vi "Reopen Files.vi"(8 "error in (no error)":errorcluster, 11 "Frame Grabber Data In":T2={"Camera Session"="", "Frame"=refnum, "AVI Refnum"=refnum, "Codecs"=[], "Frame number"=0, "Tracking File Refnum"=refnum, "Tick Count"=0, "Probe Object"=refnum, "Playback Probe Data"=[], "Rigid Body"={"Position"={"x (mm)"=0.0, "y (mm)"=0.0, "z (mm)"=0.0}, "Orientation"={"Pitch (rad)"=0.0, "Yaw (rad)"=0.0, "Roll (rad)"=0.0}, "Quaternion"={"qx"=0.0, "qy"=0.0, "qz"=0.0, "qw"=0.0}, "Tracked?"=FALSE}, "Total no frames playback"=0, "Video FPS"=0.0, "Camera connected?"=FALSE, "Scene"=refnum, "Cropped Frame"=refnum, "Tracker FPS"=0.0, "Crop ROI"=[], "Presentation Values"=[], "Elapsed time (ms)"=0, "Camera frames playback"=0, "Refnums"={"Live Refnum"=refnum, "Record Refnum"=refnum, "Playback Refnum"=refnum, "Frame Slider Refnum"=refnum, "Pause Refnum"=refnum, "Home Refnum"=refnum, "Set Crop Refnum"=refnum, "Clear Crop Refnum"=refnum, "stop refnum"=refnum, "Playback Rate Refnum"=refnum, "Presentation Refnum"=refnum, "Crop Time Frame Slider Refnum"=refnum, "Cancel Save Refnum"=refnum, "Reverse Playback Refnum"=refnum, "Recording Settings Refnum"=refnum, "Continuous Playback Refnum"=refnum, "Annotation Refnum"=refnum, "Export All Refnum"=refnum, "Export List Refnum"=refnum, "Fill List Refnum"=refnum, "Save Crop Refnum"=refnum, "Skip Forward Refnum"=refnum, "Skip Backward Refnum"=refnum, "Single Annotation Refnum"=refnum, "Load Video Refnum"=refnum, "Set Start Refnum"=refnum, "Set End Refnum"=refnum, "Add to List Refnum"=refnum, "List of Annotations Refnum"=refnum, "Camera Frame Refnum"=refnum, "Load Image Refnum"=refnum, "Saving Refnum"=refnum}, "Dimensions"={"Probe Dimensions"={"Probe Width"=0.0, "Probe Depth"=0.0, "Probe Height"=0.0}, "Room Dimensions"={"Room Width"=0.0, "Room Depth"=0.0, "Room Height"=0.0}}, "Playback Data As Strings"=[], "Cropped Tracking File Refnum"=refnum, "Cropped AVI Refnum"=refnum, "Header"=[], "Total euclidian distance"=0.0, "Annotation File Path"=path "", "Playback File Path"=path "", "Size per frame"=0.0, "Ground Truth File Refnum"=refnum, "Annotation Array"=[], "Annotation TIFFs Folder"=path "", "overwriting open file?"=FALSE, "Image Sequence"=[], "Video/Image Flag"=enum."Playback Video Frame", "Image sequence?"=FALSE, "Image sequence filenames"=[], "Mask"=refnum, "Crop Type"=enum."Rectangle"}) -> (0 "error out":errorcluster, 1 "Playback video path":path, 2 "Annotation List":T1[](array[typedef]) {"Frame Start" min=0}, 3 "Frame Grabber Data Out":T2={"Camera Session"="", "Frame"=refnum, "AVI Refnum"=refnum, "Codecs"=[], "Frame number"=0, "Tracking File Refnum"=refnum, "Tick Count"=0, "Probe Object"=refnum, "Playback Probe Data"=[], "Rigid Body"={"Position"={"x (mm)"=0.0, "y (mm)"=0.0, "z (mm)"=0.0}, "Orientation"={"Pitch (rad)"=0.0, "Yaw (rad)"=0.0, "Roll (rad)"=0.0}, "Quaternion"={"qx"=0.0, "qy"=0.0, "qz"=0.0, "qw"=0.0}, "Tracked?"=FALSE}, "Total no frames playback"=0, "Video FPS"=0.0, "Camera connected?"=FALSE, "Scene"=refnum, "Cropped Frame"=refnum, "Tracker FPS"=0.0, "Crop ROI"=[], "Presentation Values"=[], "Elapsed time (ms)"=0, "Camera frames playback"=0, "Refnums"={"Live Refnum"=refnum, "Record Refnum"=refnum, "Playback Refnum"=refnum, "Frame Slider Refnum"=refnum, "Pause Refnum"=refnum, "Home Refnum"=refnum, "Set Crop Refnum"=refnum, "Clear Crop Refnum"=refnum, "stop refnum"=refnum, "Playback Rate Refnum"=refnum, "Presentation Refnum"=refnum, "Crop Time Frame Slider Refnum"=refnum, "Cancel Save Refnum"=refnum, "Reverse Playback Refnum"=refnum, "Recording Settings Refnum"=refnum, "Continuous Playback Refnum"=refnum, "Annotation Refnum"=refnum, "Export All Refnum"=refnum, "Export List Refnum"=refnum, "Fill List Refnum"=refnum, "Save Crop Refnum"=refnum, "Skip Forward Refnum"=refnum, "Skip Backward Refnum"=refnum, "Single Annotation Refnum"=refnum, "Load Video Refnum"=refnum, "Set Start Refnum"=refnum, "Set End Refnum"=refnum, "Add to List Refnum"=refnum, "List of Annotations Refnum"=refnum, "Camera Frame Refnum"=refnum, "Load Image Refnum"=refnum, "Saving Refnum"=refnum}, "Dimensions"={"Probe Dimensions"={"Probe Width"=0.0, "Probe Depth"=0.0, "Probe Height"=0.0}, "Room Dimensions"={"Room Width"=0.0, "Room Depth"=0.0, "Room Height"=0.0}}, "Playback Data As Strings"=[], "Cropped Tracking File Refnum"=refnum, "Cropped AVI Refnum"=refnum, "Header"=[], "Total euclidian distance"=0.0, "Annotation File Path"=path "", "Playback File Path"=path "", "Size per frame"=0.0, "Ground Truth File Refnum"=refnum, "Annotation Array"=[], "Annotation TIFFs Folder"=path "", "overwriting open file?"=FALSE, "Image Sequence"=[], "Video/Image Flag"=enum."Playback Video Frame", "Image sequence?"=FALSE, "Image sequence filenames"=[], "Mask"=refnum, "Crop Type"=enum."Rectangle"}, 4 "Both exist and open?":bool, 5 "Number of Video Frames":u32, 7 "Number of Tracker Frames":u32)   [LabVIEW 2017]
uses:
  Controls/Frame Grabber Data.ctl
  <vilib>/userdefined/High Color/IMAQdx.ctl
  <vilib>/vision/Image Controls.llb/IMAQ Image.ctl
  <vilib>/vision/Avi.llb/IMAQ AVI2 Refnum.ctl
  Controls/Rigid Body Info.ctl
  Controls/Position.ctl
  Controls/Orientation.ctl
  Controls/Refnums.ctl
  Controls/Recording Settings.ctl
  Controls/Operator Settings.ctl
  Controls/Operator.ctl
  Controls/Patient Settings.ctl
  Controls/Dimensions.ctl
  Controls/Room Dimensions.ctl
  Controls/Crop Video State.ctl
  Controls/Crop Type.ctl
  Controls/Annotation Sequence Details.ctl
  <vilib>/Utility/file.llb/Read Delimited Spreadsheet (string).vi
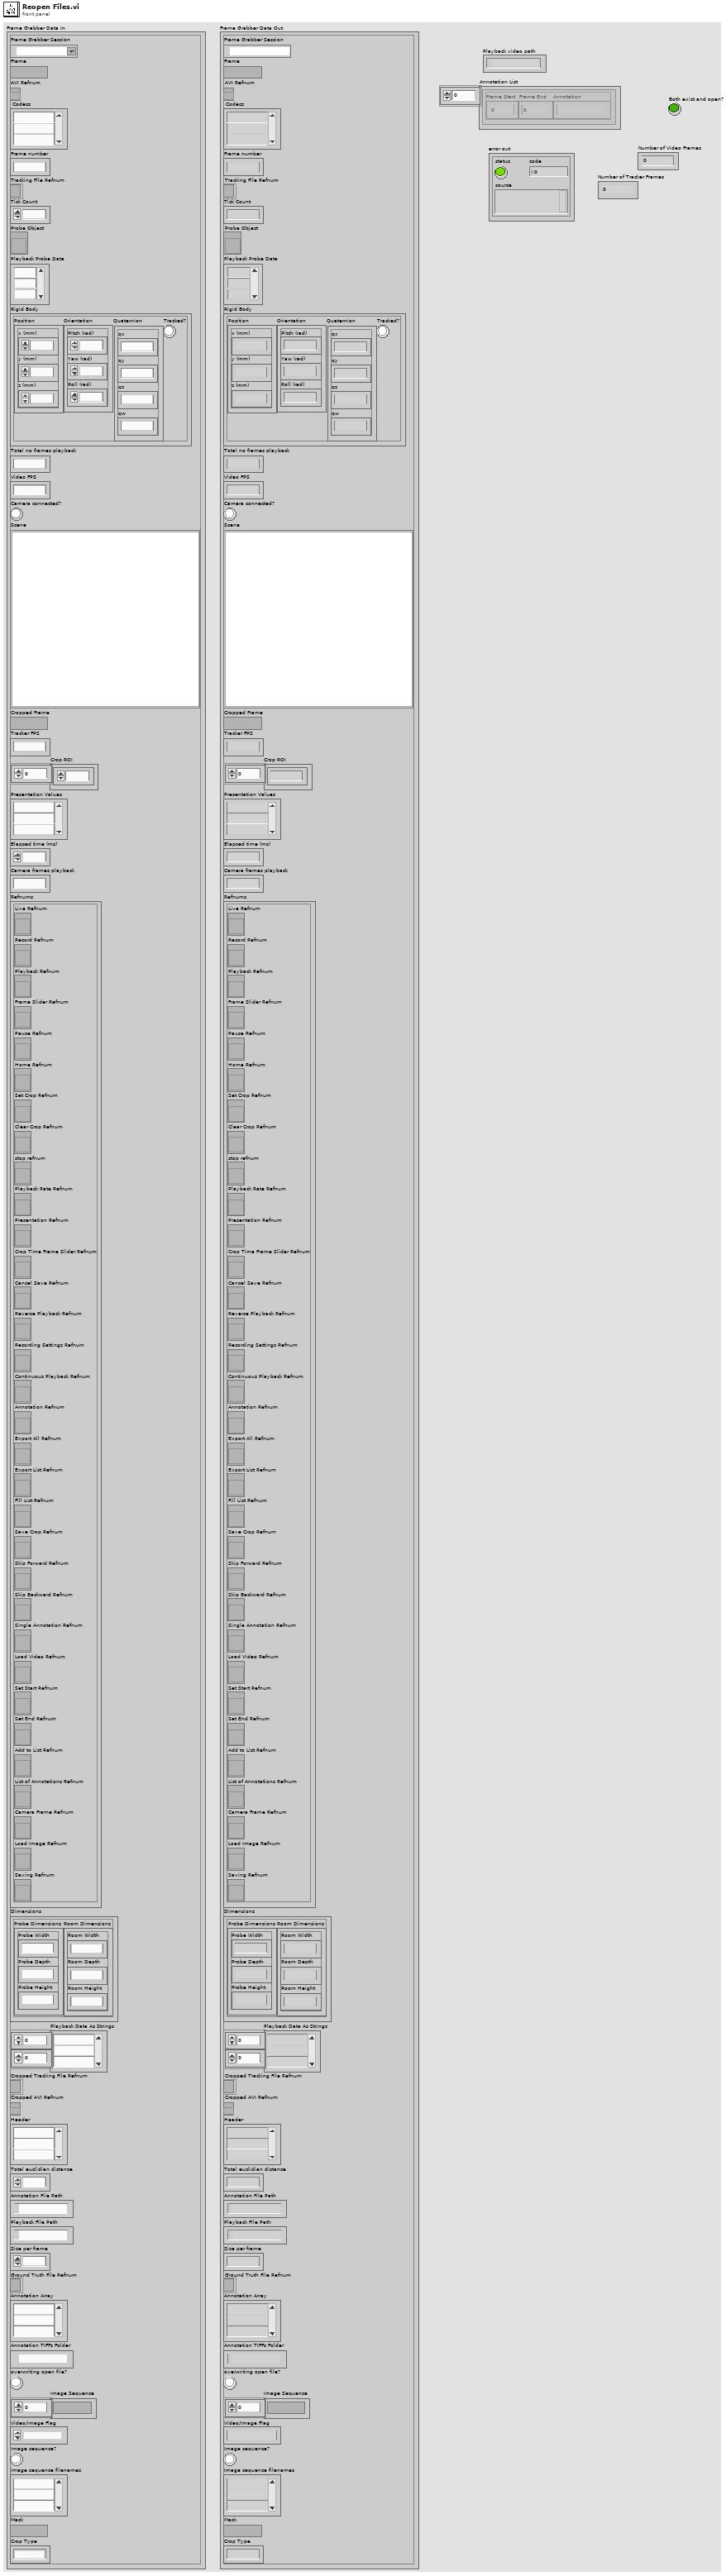
[diagram p1: front panel]
types:
  T1 = typedef "Annotation Sequence Details.ctl" = cluster{"Frame Start":i32, "Frame End":i32, "Annotation":string}
  T2 = typedef "Frame Grabber Data.ctl" = cluster{"Camera Session":T3, "Frame":T4, "AVI Refnum":T5, "Codecs":string[], "Frame number":u32, "Tracking File Refnum":refnum<file>, "Tick Count":u32, "Probe Object":refnum<vi>, "Playback Probe Data":dbl[][], "Rigid Body":T6, "Total no frames playback":i32, "Video FPS":dbl, "Camera connected?":bool, "Scene":refnum<vi>, "Cropped Frame":T4, "Tracker FPS":dbl, "Crop ROI":i32[], "Presentation Values":string[], "Elapsed time (ms)":u32, "Camera frames playback":u32, "Refnums":T9, "Dimensions":T10, "Playback Data As Strings":string[][], "Cropped Tracking File Refnum":refnum<file>, "Cropped AVI Refnum":T5, "Header":string[], "Total euclidian distance":dbl, "Annotation File Path":path, "Playback File Path":path, "Size per frame":dbl, "Ground Truth File Refnum":refnum<file>, "Annotation Array":string[], "Annotation TIFFs Folder":path, "overwriting open file?":bool, "Image Sequence":T4[], "Video/Image Flag":T12, "Image sequence?":bool, "Image sequence filenames":string[], "Mask":T4, "Crop Type":T13}
  T3 = typedef "IMAQdx.ctl" = refnum<k21>
  T4 = typedef "IMAQ Image.ctl" = refnum<image>
  T5 = typedef "IMAQ AVI2 Refnum.ctl" = refnum<k20>
  T6 = typedef "Rigid Body Info.ctl" = cluster{"Position":T7, "Orientation":T8, "Quaternion":cluster{"qx":sgl, "qy":sgl, "qz":sgl, "qw":sgl}, "Tracked?":bool}
  T7 = typedef "Position.ctl" = cluster{"x (mm)":sgl, "y (mm)":sgl, "z (mm)":sgl}
  T8 = typedef "Orientation.ctl" = cluster{"Pitch (rad)":sgl, "Yaw (rad)":sgl, "Roll (rad)":sgl}
  T9 = typedef "Refnums.ctl" = cluster{"Live Refnum":refnum<vi>, "Record Refnum":refnum<vi>, "Playback Refnum":refnum<vi>, "Frame Slider Refnum":refnum<vi>, "Pause Refnum":refnum<vi>, "Home Refnum":refnum<vi>, "Set Crop Refnum":refnum<vi>, "Clear Crop Refnum":refnum<vi>, "stop refnum":refnum<vi>, "Playback Rate Refnum":refnum<vi>, "Presentation Refnum":refnum<vi>, "Crop Time Frame Slider Refnum":refnum<vi>, "Cancel Save Refnum":refnum<vi>, "Reverse Playback Refnum":refnum<vi>, "Recording Settings Refnum":refnum<vi>, "Continuous Playback Refnum":refnum<vi>, "Annotation Refnum":refnum<vi>, "Export All Refnum":refnum<vi>, "Export List Refnum":refnum<vi>, "Fill List Refnum":refnum<vi>, "Save Crop Refnum":refnum<vi>, "Skip Forward Refnum":refnum<vi>, "Skip Backward Refnum":refnum<vi>, "Single Annotation Refnum":refnum<vi>, "Load Video Refnum":refnum<vi>, "Set Start Refnum":refnum<vi>, "Set End Refnum":refnum<vi>, "Add to List Refnum":refnum<vi>, "List of Annotations Refnum":refnum<vi>, "Camera Frame Refnum":refnum<vi>, "Load Image Refnum":refnum<vi>, "Saving Refnum":refnum<vi>}
  T10 = typedef "Dimensions.ctl" = cluster{"Probe Dimensions":cluster{"Probe Width":sgl, "Probe Depth":sgl, "Probe Height":sgl}, "Room Dimensions":T11}
  T11 = typedef "Room Dimensions.ctl" = cluster{"Room Width":dbl, "Room Depth":dbl, "Room Height":dbl}
  T12 = typedef "Crop Video State.ctl" = enum16{"Init", "Wait", "Load Image", "Load Video", "Play/Pause", "Playback Video Frame", "Display Image", "Save Image Sequence", "Save Video", "Export List", "Export All", "Close", "Set Crop Area", "Reset Crop Area", "Crop Inside", "Crop Outside", "Multi-Crop", "Re-Open Files", "Annotate Frame", "Annotate Clip", "Add to List", "Fill List", "Set Start", "Set End", "Error Handling", "Shutdown"}
  T13 = typedef "Crop Type.ctl" = enum16{"Rectangle", "Annulus"}
  T14 = enum8{"Enabled", "Disabled", "Disabled and Grayed Out"}
  T15 = cluster{"Width":u32, "Height":u32, "Frames Per Second":u32, "Codec":string, "Has Data":bool}
  T16 = cluster{"Scale.Range:Minimum":i32, "Number of Frames":u32, "Scale.Range:Minimum":i32}
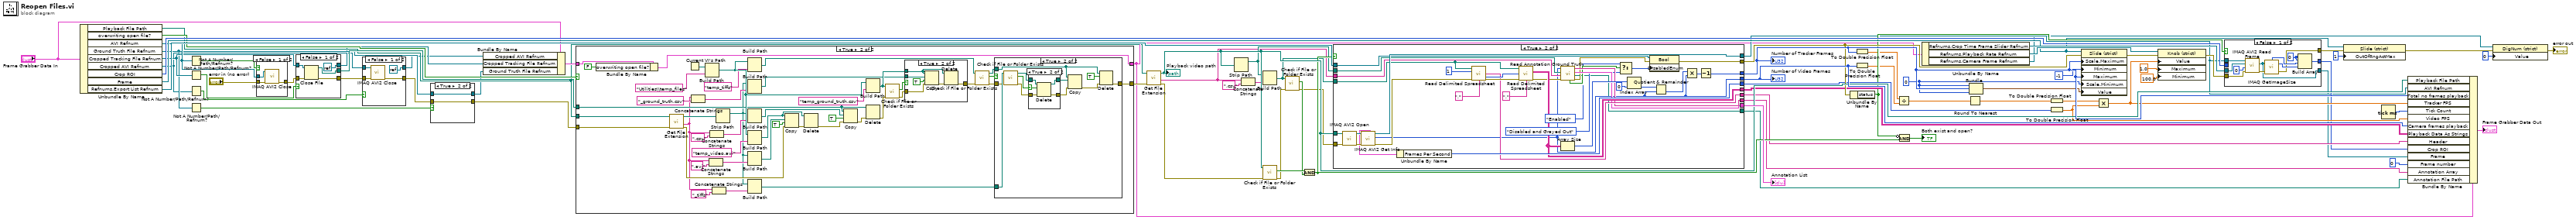
[diagram p0: block diagram]
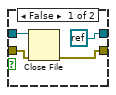
[diagram p2: hidden frame]
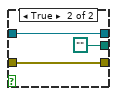
[diagram p4: hidden frame]
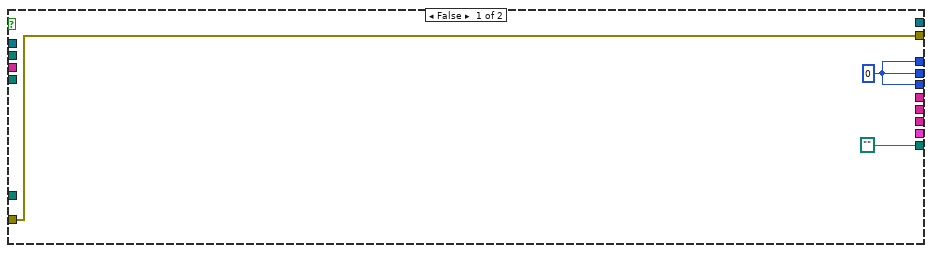
[diagram p7: hidden frame]
diagram:
  w24 = 0 ("Scale.Range:Minimum")
  n1 = Unbundle By Name("Frame Grabber Data In") -> ("Playback File Path"=w6:path, "overwriting open file?"=w7:bool, "AVI Refnum"=w15:T5, "Ground Truth File Refnum"=w5:refnum<file>, "Cropped Tracking File Refnum"=w8:refnum<file>, "Cropped AVI Refnum"=w1:T5, "Crop ROI"=w75:i32[], "Frame"=w76:T4, "Refnums.Export List Refnum"=w77:refnum<vi>)
  n2 = Not A Number/Path/Refnum?(number/path/refnum=w15) -> (NaN/Path/Refnum?=w14:bool)
  n3 = Not A Number/Path/Refnum?(number/path/refnum=w8) -> (NaN/Path/Refnum?=w10:bool)
  n4 = Not A Number/Path/Refnum?(number/path/refnum=w1) -> (NaN/Path/Refnum?=w9:bool)
  n5 = Not A Number/Path/Refnum?(number/path/refnum=w5) -> (NaN/Path/Refnum?=w11:bool)
  n6 = case shown="False" w14 {
    tunnel: [w80 w81] -> w72
    tunnel: "error in (no error)" -> [w79 w81]
    tunnel: w15 -> [w78 _]
    frame False {
      n7 = call "IMAQ AVI2 Close"("error in (no error)"=w79, "AVI Refnum"=w78) -> ("error out"=w80:errorcluster)  [unwired: 9 in]
    }
    frame True {
    }
  }
  n8 = case shown="False" w10 {
    tunnel: w8 -> [w86 w87]
    tunnel: [w85 w89] -> w74
    tunnel: w72 -> [w84 w89]
    tunnel: [w83 path ""] -> w16
    tunnel: [refnum<k0> refnum w87] -> w4
    frame False {
      n9 = Close File(refnum=w86, error in=w84) -> (path=w83:path, error out=w85:errorcluster)
    }
    frame True {
    }
  }
  n10 = case shown="False" w9 {
    tunnel: w1 -> [w93 w94]
    tunnel: w74 -> [w92 w95]
    tunnel: [w91 w95] -> w13
    tunnel: [refnum<k0> refnum w94] -> w3
    frame False {
      n11 = call "IMAQ AVI2 Close"("error in (no error)"=w92, "AVI Refnum"=w93) -> ("error out"=w91:errorcluster)  [unwired: 9 in]
    }
    frame True {
    }
  }
  n12 = case shown="True" w11 {
    tunnel: [w99 w101] -> w12
    tunnel: w13 -> [w98 w101]
    tunnel: w5 -> [w97 w100]
    tunnel: [refnum<k0> refnum w100] -> w2
    frame False {
      n13 = Close File(refnum=w97, error in=w98) -> (error out=w99:errorcluster)  [unwired: 1 out]
    }
    frame True {
    }
  }
  n14 = Bundle By Name(cluster="Frame Grabber Data In", "Cropped AVI Refnum"=w3, "Cropped Tracking File Refnum"=w4, "Ground Truth File Refnum"=w2) -> (w18:T2)
  n15 = case shown="True" w7 {
    tunnel: w18 -> [w103 w147]
    tunnel: [w103 w144] -> w19
    tunnel: [w102 w125] -> w71
    tunnel: w12 -> [w102 w119]
    tunnel: w6 -> [_ w136]
    tunnel: w16 -> [_ w135]
    frame False {
    }
    frame True {
      n16 = Bundle By Name(cluster=w147, "overwriting open file?"=FALSE) -> (w144:T2)
      n17 = call <vilib>:"Get File Extension.vi"("error in (no error)"=w119, "file"=w136) -> ("error out"=w120:errorcluster, "filename without extension"=w106:string, "dup file"=w122:path)  [unwired: 5 in, 2 out]
      n18 = Current VI's Path() -> (path=w142:path)
      n19 = Concatenate Strings(w106, "_ground_truth.csv" ("string")) -> (w111:string)
      n20 = Build Path(base path=w142, name or relative path="Utilities\\temp_files") -> (appended path=w143:path)
      n21 = Concatenate Strings(w106, ".avi" ("string")) -> (w115:string)
      n22 = Concatenate Strings(w106, ".csv" ("string")) -> (w121:string)
      n23 = Concatenate Strings(w106, "_tiffs" ("string")) -> (w107:string)
      n24 = Strip Path(path=w122) -> (stripped path=w105:path)  [unwired: 1 out]
      n25 = Build Path(base path=w143, name or relative path="temp_tiffs") -> (appended path=w133:path)
      n26 = Build Path(base path=w105, name or relative path=w111) -> (appended path=w109:path)
      n27 = Build Path(base path=w105, name or relative path=w121) -> (appended path=w117:path)
      n28 = Build Path(base path=w143, name or relative path="temp_video.avi") -> (appended path=w118:path)
      n29 = Build Path(base path=w105, name or relative path=w115) -> (appended path=w114:path)
      n30 = Build Path(base path=w105, name or relative path=w107) -> (appended path=w104:path)
      n31 = Copy(8:w120, 9:TRUE ("overwrite (F)"), 10:w114, 11:w118) -> (0:w134:errorcluster)  [unwired: 1 in, 2 out]
      n32 = Delete(path (use dialog)=w118, error in=w134) -> (error out=w132:errorcluster)  [unwired: 3 in, 2 out]
      n33 = Copy(8:w132, 9:TRUE ("overwrite (F)"), 10:w117, 11:w135) -> (0:w145:errorcluster)  [unwired: 1 in, 2 out]
      n34 = Build Path(base path=w143, name or relative path="temp_ground_truth.csv") -> (appended path=w129:path)
      n35 = Delete(path (use dialog)=w135, error in=w145) -> (error out=w131:errorcluster)  [unwired: 3 in, 2 out]
      n36 = call <vilib>:"Check if File or Folder Exists.vi"("error in (no error)"=w131, "path"=w129) -> ("error out"=w130:errorcluster, "file or folder exists?"=w128:bool)  [unwired: 7 in, 1 out]
      n37 = case shown="True" w128 {
        tunnel: w130 -> [w167 w173]
        tunnel: w129 -> [_ w170]
        tunnel: [w167 w171] -> w127
        tunnel: w109 -> [_ w168]
        frame False {
        }
        frame True {
          n38 = Copy(8:w173, 9:TRUE ("overwrite (F)"), 10:w168, 11:w170) -> (0:w172:errorcluster)  [unwired: 1 in, 2 out]
          n39 = Delete(path (use dialog)=w170, error in=w172) -> (error out=w171:errorcluster)  [unwired: 3 in, 2 out]
        }
      }
      n40 = call <vilib>:"Check if File or Folder Exists.vi"("error in (no error)"=w127, "path"=w133) -> ("error out"=w126:errorcluster, "file or folder exists?"=w124:bool, "dup path"=w123:path)  [unwired: 7 in]
      n41 = case shown="True" w124 {
        tunnel: w126 -> [w148 w154]
        tunnel: w123 -> [_ w157]
        tunnel: [w148 w158] -> w125
        tunnel: w104 -> [_ w155]
        frame False {
        }
        frame True {
          n42 = call <vilib>:"Check if File or Folder Exists.vi"("error in (no error)"=w154, "path"=w155) -> ("error out"=w153:errorcluster, "file or folder exists?"=w152:bool, "dup path"=w151:path)  [unwired: 7 in]
          n43 = case shown="True" w152 {
            selector: w152 -> [_ w165]
            tunnel: w153 -> [w161 w166]
            tunnel: w151 -> [w160 w164]
            tunnel: [w161 w163] -> w150
            tunnel: [w160 w162] -> w149
            frame False {
            }
            frame True {
              n44 = Delete(path (use dialog)=w164, entire hierarchy (F)=w165, error in=w166) -> (deleted path=w162:path, error out=w163:errorcluster)  [unwired: 2 in, 1 out]
            }
          }
          n45 = Copy(8:w150, 10:w149, 11:w157) -> (0:w159:errorcluster)  [unwired: 2 in, 2 out]
          n46 = Delete(path (use dialog)=w157, entire hierarchy (F)=TRUE, error in=w159) -> (error out=w158:errorcluster)  [unwired: 2 in, 2 out]
        }
      }
    }
  }
  n47 = call <vilib>:"Get File Extension.vi"("error in (no error)"=w71, "file"=w6) -> ("error out"=w58:errorcluster, "filename without extension"=w25:string, "dup file"=w64:path)  [unwired: 5 in, 2 out]
  "Playback video path" <- w64
  n48 = Strip Path(path=w64) -> (stripped path=w26:path)  [unwired: 1 out]
  n49 = Concatenate Strings(w25, ".csv" ("string")) -> (w20:string)
  n50 = Build Path(base path=w26, name or relative path=w20) -> (appended path=w56:path)
  n51 = call <vilib>:"Check if File or Folder Exists.vi"("error in (no error)"=w58, "path"=w64) -> ("error out"=w54:errorcluster, "file or folder exists?"=w57:bool)  [unwired: 7 in, 1 out]
  n52 = call <vilib>:"Check if File or Folder Exists.vi"("error in (no error)"=w54, "path"=w56) -> ("error out"=w28:errorcluster, "file or folder exists?"=w55:bool)  [unwired: 7 in, 1 out]
  n53 = And(x=w57, y=w55) -> (x .and. y?=w63:bool)
  n54 = case shown="True" w63 {
    tunnel: w28 -> [w176 w191]
    tunnel: w64 -> [_ w212]
    tunnel: [w176 w182] -> w61
    tunnel: [_ w209] -> w40
    tunnel: w56 -> [_ w204]
    tunnel: [w175 w187] -> w67
    tunnel: [w175 w207] -> w59
    tunnel: [w175 w185] -> w69
    tunnel: [_ w201] -> w45
    tunnel: [_ w197] -> w44
    tunnel: [_ w195] -> w70
    tunnel: [_ w194] -> w27
    tunnel: w26 -> [_ w193]
    tunnel: w25 -> [_ w192]
    tunnel: w77 -> [_ w184]
    tunnel: [path "" w177] -> w22
    frame False {
      w175 = 0 ("Number of Frames")
    }
    frame True {
      n55 = call "IMAQ AVI2 Open"("error in (no error)"=w191, "AVI File Path"=w212) -> ("error out"=w211:errorcluster, "AVI Refnum"=w210:T5)  [unwired: 8 in]
      n56 = call "IMAQ AVI2 Get Info"("error in (no error)"=w211, "AVI Refnum"=w210) -> ("error out"=w206:errorcluster, "Number of Frames"=w187:u32, "AVI Refnum (duplicate)"=w209:T5, "Frame Data"=w208:T15)  [unwired: 5 in, 1 out]
      n57 = Unbundle By Name(w208) -> ("Frames Per Second"=w207:u32)
      n58 = call-poly <vilib>:"Read Delimited Spreadsheet.vi"("file path (dialog if empty)"=w204, "number of rows (all:-1)"=1, "error in (no error)"=w206, "delimiter (\\t)"="," ("delimiter (\\t)")) -> ("first row"=w197:string[], "mark after read (chars.)"=w202:i32, "error out"=w203:errorcluster)  [unwired: 6 in, 3 out]
      n59 = call-poly <vilib>:"Read Delimited Spreadsheet.vi"("file path (dialog if empty)"=w204, "start of read offset (chars.:0)"=w202, "error in (no error)"=w203, "delimiter (\\t)"="," ("delimiter (\\t)")) -> ("all rows"=w201:string[][], "error out"=w190:errorcluster)  [unwired: 6 in, 4 out]
      n60 = Array Size(array=w201) -> (size(s)=w200:i32[])
      n61 = call "Read Annotation Ground Truth.vi"("Error In"=w190, "Filename without extension"=w192, "Folder"=w193, "Total no frames playback"=w187) -> ("Error Out"=w183:errorcluster, "annotation file path"=w177:path, "Annotation List"=w195:T1[], "Annotation array (strings)"=w194:string[], "annotation list exists?"=w181:bool)  [unwired: 3 in]
      n62 = Select(t=T14."Enabled" ("Disabled"), s=w181, f=T14."Disabled and Grayed Out") -> (s? t:f=w179:T14)
      n63 = Index Array(array=w200, index=0) -> (element=w189:i32)
      n64 = property class="Bool"(reference=w184, error in=w183, "DisabledEnum"=w179) -> (error out=w182:errorcluster)  [unwired: 1 out]
      n65 = Quotient & Remainder(x=w189, y=w187) -> (floor(x/y)=w188:u32)  [unwired: 1 out]
      n66 = Multiply(x=w188, y=w187) -> (x*y=w186:u32)
      n67 = Decrement(x=w186) -> (x-1=w185:u32)
    }
  }
  "Annotation List" <- w70
  "Number of Tracker Frames" <- w69
  "Number of Video Frames" <- w67
  n68 = Unbundle By Name(w61) -> ("status"=w43:bool)
  n69 = To Double Precision Float(number=w69) -> (double precision float=w37:dbl)
  n70 = To Double Precision Float(number=w67) -> (double precision float=w36:dbl)
  n71 = Divide(x=w37, y=w36) -> (x/y=w60:dbl)
  n72 = Compound Arithmetic op=AND(invert w43, w63) -> (→"Both exist and open?":bool)
  n73 = Unbundle By Name(w19) -> ("Refnums.Crop Time Frame Slider Refnum"=w33:refnum<vi>, "Refnums.Playback Rate Refnum"=w53:refnum<vi>, "Refnums.Camera Frame Refnum"=w30:refnum<vi>)
  n74 = Round To Nearest(number=w60) -> (nearest integer value=w38:dbl)
  n75 = Bundle("Scale.Range:Minimum"=w24, "Number of Frames"=w69, "Scale.Range:Minimum"=w24) -> (w46:T16)  [unwired: 1 in]
  n76 = To Double Precision Float(number=w38) -> (double precision float=w47:dbl)
  n77 = To Double Precision Float(number=w59) -> (double precision float=w48:dbl)
  n78 = property class="Slide (strict)"(reference=w33, error in=w61, "Scale.Maximum"=w69, "Minimum"=-1 ("Scale.Range:Minimum"), "Maximum"=w69, "Scale.Minimum"=w24, "Value"=w46) -> (error out=w51:errorcluster)  [unwired: 1 out]
  n79 = Multiply(x=w47, y=w48) -> (x*y=w52:dbl)
  n80 = property class="Knob (strict)"(reference=w53, error in=w51, "Value"=w52, "Maximum"=1.0 ("Data Entry Limits:Maximum"), "Minimum"=100.0 ("Data Entry Limits:Minimum")) -> (error out=w42:errorcluster)  [unwired: 1 out]
  n81 = case shown="False" w43 {
    tunnel: w42 -> [w223 w225]
    tunnel: w75 -> [_ w226]
    tunnel: [w218 w226] -> w41
    tunnel: w40 -> [w217 _]
    tunnel: w76 -> [w215 w224]
    tunnel: [w214 w225] -> w34
    tunnel: [w213 w224] -> w39
    frame False {
      w219 = 0 ("element")
      n82 = call "IMAQ AVI2 Read Frame"("error in (no error)"=w223, "Frame Number"=u32 0, "Image"=w215, "AVI Refnum"=w217) -> ("error out"=w222:errorcluster, "Image Out"=w213:T4)  [unwired: 5 in, 1 out]
      n83 = call "IMAQ GetImageSize"("Image"=w213, "error in (no error)"=w222) -> ("Y Resolution"=w221:i32, "X Resolution"=w220:i32, "error out"=w214:errorcluster)  [unwired: 2 in]
      n84 = Build Array(w219, w219, w220, w221) -> (w218:i32[])
    }
    frame True {
    }
  }
  n85 = property class="Slide (strict)"(reference=w33, error in=w34, "OutOfRngActMax"=u8 1 ("Response to Value Outside Limits:Maximum")) -> (error out=w31:errorcluster)  [unwired: 1 out]
  n86 = Tick Count (ms)() -> (millisecond timer value=w62:u32)
  n87 = Bundle By Name(cluster=w19, "Playback File Path"=w64, "AVI Refnum"=w40, "Total no frames playback"=w69, "Tracker FPS"=w52, "Tick Count"=w62, "Video FPS"=w48, "Camera frames playback"=w67, "Playback Data As Strings"=w45, "Header"=w44, "Crop ROI"=w41, "Frame"=w39, "Frame number"=u32 0, "Annotation Array"=w27, "Annotation File Path"=w22) -> (→"Frame Grabber Data Out":T2)
  n88 = property class="DigNum (strict)"(reference=w30, error in=w31, "Value"=u32 0) -> (error out=→"error out":errorcluster)  [unwired: 1 out]
